vi "MON_LS218_Init.vi"(0 "error in (no error)":errorcluster, 1 "found VISA":refnum<visa-resource-name>) -> (2 "error out":errorcluster, 3 "Reply":string, 4 "VISA Out":refnum<visa-resource-name>)   [LabVIEW 2012]
uses:
  Common/Call-VISA-Close.ctl
  <instrlib>/Lake Shore Cryotronics 218/Lake Shore Cryotronics 218.lvlib
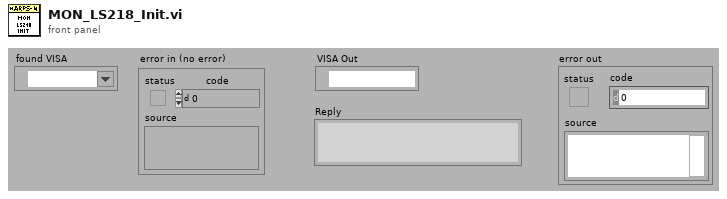
[diagram p1: front panel]
types:
  T1 = typedef "Call-VISA-Close.ctl" = enum16{"DON'T CALL", "CALL CLOSE"}
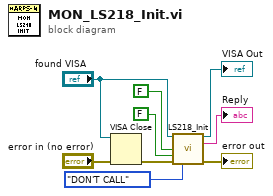
[diagram p0: block diagram]
diagram:
  n1 = VISA Close(VISA resource name="found VISA", error in (no error)="error in (no error)") -> (error out=w9:errorcluster)
  n2 = call "LS218_Init.vi"("VISA"="found VISA", "Reset (T: Reset)"=FALSE ("Don't Reset"), "Reset Defaults (F:Dont Reset)"=FALSE, "error in (no error)"=w9, "call-VISA-Close"=Call-VISA-Close."DON'T CALL") -> ("VISA Out"=→"VISA Out":refnum<visa-resource-name>, "Reply"=→"Reply":string, "error out"=→"error out":errorcluster)  [unwired: 8 in]
